vi "DAQmx Create Channel (CI-Frequency).vi"(0 "task in":refnum<k21>, 1 "maximum value":dbl=100.0 format="%0.6f", 2 "minimum value":dbl=2.0 format="%0.6f", 3 "measurement method":i32(ring)=10105 items=["Low Frequency with 1 Counter"=10105, "High Frequency with 2 Counters"=10157, "Large Range with 2 Counters"=10205], 5 "counter":tag, 6 "divisor":u32=4, 7 "name to assign":string, 9 "units":i32(ring)=10373 items=["Hz"=10373, "Ticks"=10304, "From Custom Scale"=10065], 11 "error in":errorcluster, 12 "custom scale name":tag, 13 "starting edge":i32(ring)=10280 items=["Rising"=10280, "Falling"=10171], 14 "measurement time":dbl=0.001 format="%0.6f") -> (4 "task out":refnum<k21>, 15 "error out":errorcluster)   [LabVIEW 2011]
doc: "Creates a channel to measure the frequency of a digital signal. You can create only one counter input channel at a time with this VI because a task can contain only one counter input channel. To read from multiple counters simultaneously, use a separate task for each counter. Connect the input signal to the default input terminal of the counter unless you select a different input terminal."
uses:
  C:/Program Files/National Instruments/LabVIEW 2011/resource/objmgr/daqmx.rc
panel:
  # "input limits"
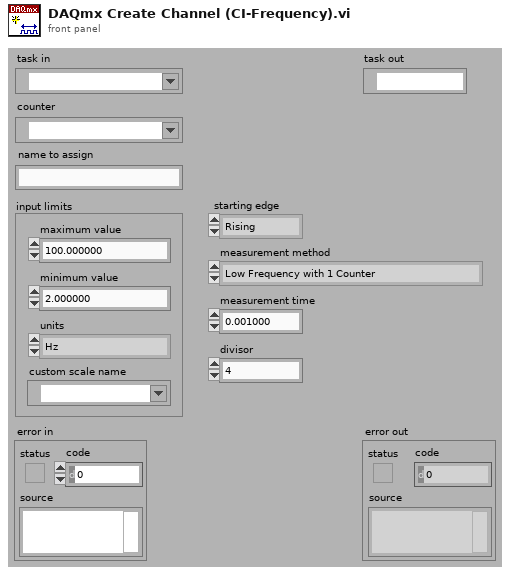
[diagram p1: front panel]
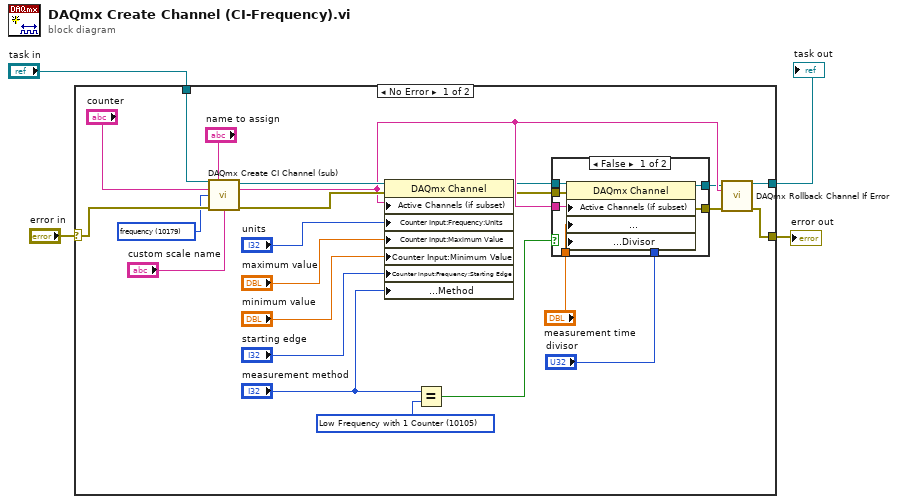
[diagram p0: block diagram]
diagram:
  n1 = case shown="No Error" "error in" {
    selector: "error in" -> [w26 w38]
    tunnel: "task in" -> [w28 w39]
    tunnel: [w16 w39] -> w2
    tunnel: [w15 w38] -> w1
    frame No Error {
      w7 = 10105 items=["Low Frequency with 1 Counter"=10105, "High Frequency with 2 Counters"=10157, "Large Range with 2 Counters"=10205] ("measurement method")
      w20 = 10179 items=["count events"=10125, "frequency"=10179, "period"=10256, "pulse width"=10267, "semi period"=10289] ("measurement type")
      n2 = call "DAQmx Create CI Channel (sub).vi"("task in"=w28, "virtual channel name"="name to assign", "physical channel name"="counter", "measurement type"=w20, "error in"=w26, "custom scale"="custom scale name") -> ("task out"=w17:refnum<k21>, "channel names"=w14:string, "error out"=w25:errorcluster)  [unwired: 7 out]
      n3 = property class="DAQmx Channel"(reference=w17, error in=w25, "Active Channels (if subset)"=w14, "Counter Input:Frequency:Units"="units", "Counter Input:Maximum Value"="maximum value", "Counter Input:Minimum Value"="minimum value", "Counter Input:Frequency:Starting Edge"="starting edge", "Counter Input:Frequency:Measurement Specifications:Method"="measurement method") -> (reference out=w13:refnum<k21>, error out=w12:errorcluster)
      n4 = Equal?(x="measurement method", y=w7) -> (x = y?=w5:bool)
      n5 = case shown="False" w5 {
        tunnel: w14 -> [w35 _]
        tunnel: w13 -> [w34 w37]
        tunnel: w12 -> [w33 w36]
        tunnel: [w32 w37] -> w11
        tunnel: [w31 w36] -> w10
        tunnel: "measurement time" -> [w30 _]
        tunnel: "divisor" -> [w29 _]
        frame False {
          n6 = property class="DAQmx Channel"(reference=w34, error in=w33, "Active Channels (if subset)"=w35, "Counter Input:Frequency:Measurement Specifications:High Frequency:Measurement Time"=w30, "Counter Input:Frequency:Measurement Specifications:Large Range:Divisor"=w29) -> (reference out=w32:refnum<k21>, error out=w31:errorcluster)
        }
        frame True {
        }
      }
      n7 = call "DAQmx Rollback Channel If Error.vi"("task in"=w11, "channel names"=w14, "error in"=w10) -> ("task out"=w16:refnum<k21>, "error out"=w15:errorcluster)  [unwired: 11 out]
    }
    frame Error {
    }
  }
  "error out" <- w1
  "task out" <- w2
